vi "countrate.vi"() -> ()   [LabVIEW 2015]
uses:
  <vilib>/Platform/TimedLoop/XDataNode/timing_clust.ctl
  <vilib>/Platform/TimedLoop/XDataNode/nitl_modes.ctl
  <vilib>/Platform/TimedLoop/XDataNode/wakeup.ctl
  <vilib>/platform/TimedLoop/XDataNode/XDataNode.xnode
  <vilib>/Platform/TimedLoop/XDataNode/XDNodeRunTimeDep.lvlib
panel:
  in  "Total Time (s)":dbl
  in  "Period (ms)":i64=1000
  out "XY Graph":cluster{dbl[], i32[]}(graph)
  out "counts per second":dbl(knob) scale=0.0..100.0
  in  "stop":bool
  # "Demo count rate VI for Physics 434"
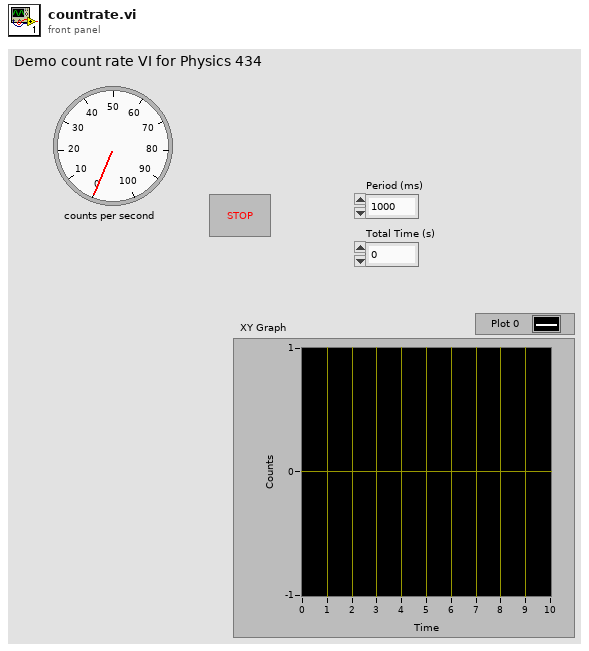
[diagram p1: front panel]
types:
  T1 = typedef "XDNodeRunTimeDep.lvlib/timing_clust.ctl" = cluster{"Expected End [f-1]":u64, "Actual End [f-1]":u64, "Finished Late? [f-1]":bool, "Expected End [i-1]":u64, "Actual End [i-1]":u64, "Finished Late? [i-1]":bool, "Expected Start [i]":u64, "Actual Start [i]":u64, "Expected Start [f]":u64, "Actual Start [f]":u64, "Source Name":string, "Structure Name":string, "Period":i64, "Deadline":i64, "Offset":i64, "Start":i64, "Priority":i32, "Timeout":i32, "Mode":T2, "Wakeup Reason":T3, "Error":errorcluster, "Source Type":string, "Secondary Source Type":string, "Global End Time":u64, "Global Start Time":u64, "Frame Duration":u64, "Iteration Duration":u64, "Assigned CPU":i32, "I/O Scan Engine Mode":u32}
  T2 = typedef "XDNodeRunTimeDep.lvlib/nitl_modes.ctl" = enum32{"No Change", "Process missed periods, maintain original phase", "Discard missed periods, maintain original phase", "Process missed periods, ignore original phase", "Discard missed periods, ignore original phase"}
  T3 = typedef "XDNodeRunTimeDep.lvlib/wakeup.ctl" = enum32{"Normal", "Aborted", "Asynchronous wakeup", "Timing source error", "Timed loop error", "Timeout"}
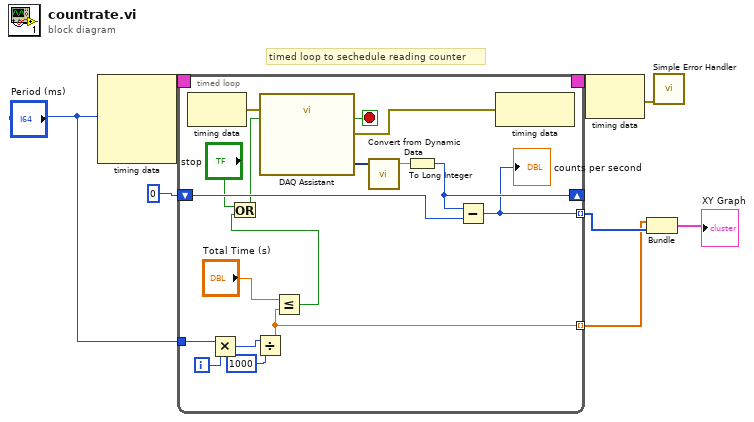
[diagram p0: block diagram]
diagram:
  # "timed loop to sechedule reading counter"
  n1 = node-c288("Period (ms)") -> (w8:T1)  [unwired: 3 in]
  n2 = timed-loop {
    timing: w8 -> [_]
    timing-out: [_] -> w7
    shift-right: [w23] -> _
    shift-left: 0 -> [w19]
    tunnel: [w18] -> w4 mode=indexing
    tunnel: "Period (ms)" -> [w12]
    tunnel: [w9] -> w2 mode=indexing
    i -> [w13]
    stop <- w24 stop-if-true
    n3 = node-c288() -> (w20:errorcluster)  [unwired: 1 in]
    n4 = Multiply(x=w12, y=w13) -> (x*y=w11:i64)
    n5 = Divide(x=w11, y=i64 1000 ("x")) -> (x/y=w9:dbl)
    n6 = Less Or Equal?(x="Total Time (s)", y=w9) -> (x <= y?=w14:bool)
    n7 = Or(x="stop", y=w14) -> (x .or. y?=w15:bool)
    n8 = call "DAQ Assistant"("error in"=w20, "stop (F)"=w15) -> ("data"=w25:dynamicdata, "stopped"=w24:bool, "error out"=w21:errorcluster)  [unwired: 14 in, 1 out]
    n9 = call "Convert from Dynamic Data"("Dynamic Data Type"=w25) -> ("Scalar"=w22:dbl)  [unwired: 3 in]
    n10 = To Long Integer(number=w22) -> (32bit integer=w23:i32)
    n11 = Subtract(x=w23, y=w19) -> (x-y=w18:i32)
    "counts per second" <- w18
    n12 = node-c288(w21) -> ()  [unwired: 1 out]
  }
  n13 = node-c288(w7) -> (w5:errorcluster)
  n14 = Bundle(w2, w4) -> (→"XY Graph":cluster{dbl[], i32[]})  [unwired: 1 in]
  n15 = call <vilib>:"Simple Error Handler.vi"("error in (no error)"=w5) -> ()  [unwired: 4 in, 5 out]
